vi "HDI-BBM Start Position Verify.vi"() -> ()   [LabVIEW 2011]
uses:
  Shared Components/Config Manager Class/Type Definitions/Part Type.ctl
  Shared Components/WorkTable Class/Type Definitions/Worktable_Mode.ctl
  Shared Components/Gantry Class/Gantry Class.lvclass
  Shared Components/WorkTable Class/WorkTable Class.lvclass
  Shared Components/Vec3d Class/Vec3d Class.lvclass
  Shared Components/Config Manager Class/Config Manager Class.lvclass
panel:
  in  "Worktable Mode":T1=enum."Gluing"
  in  "Part Type":T2
  in  "Chuck":i32
  in  "Quit":bool
  out "Current fiducial":string
  out "error out":errorcluster
  out "preview":T3(plugin-control)
  out "Current Position":cluster{"X":dbl, "Y":dbl, "Z":dbl}
  in  "Slot":i32
  in  "Next":bool
  in  "Config Folder":path=path "C:/Users/Husker/Desktop/gantry/Config"
  # "Set this to the appropriate slot number(0-3) before running"
  # "Set this to the appropriate chuck number(0-4) before running"
  # "Press this button to go to \nnext fiducial"
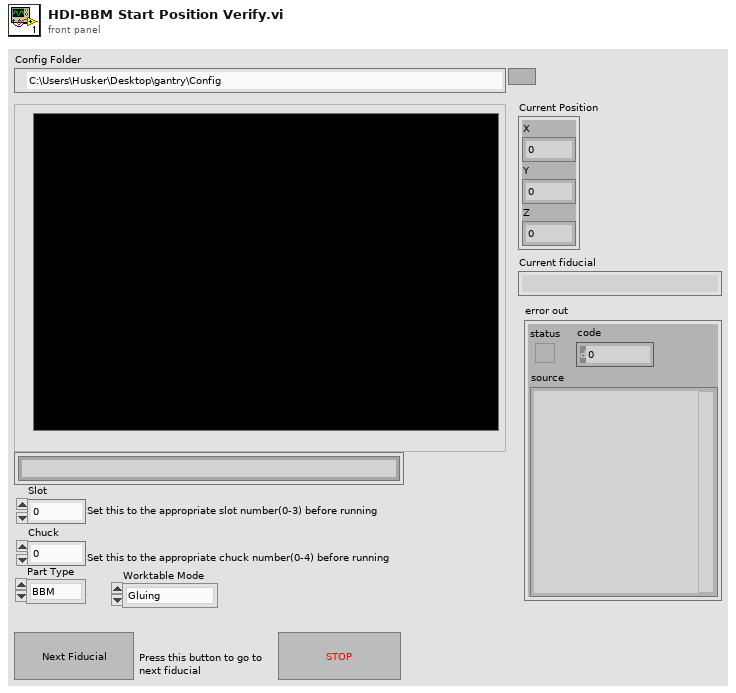
[diagram p1: front panel]
types:
  T1 = typedef "Worktable_Mode.ctl" = enum16{"Encapsulation", "Gluing"}
  T2 = typedef "Part Type.ctl" = enum16{"BBM", "HDI", "BARE HDI", "GLUERESERVOIR", "STAMP_1", "STAMP_2", "STAMP_3", "STAMP_4", "STAMP_5", "WEIGHT_1", "WEIGHT_2", "WEIGHT_3", "WEIGHT_4", "WEIGHT_5", "WEIGHT_6", "WEIGHT_7", "WEIGHT_8", "PICKER_TOOL", "GRABER_TOOL"}
  T3 = typedef "IMAQ Image.ctl" = refnum<image>
  T4 = typedef "Image Type" = u32
  T5 = typedef "Fiducial Type.ctl" = enum16{"HDI", "BBM"}
  T6 = cluster{"Feature Coordinates":refnum<class "Vec3d Class.lvclass">, "Feature Name":string}[]
  T7 = cluster{"Feature Coordinates":refnum<class "Vec3d Class.lvclass">, "Feature Name":string}
  T8 = typedef "Worktable_Module Slot.ctl" = cluster{"Slot State":enum16{"Empty", "Bare HDI", "Unglued", "Stamped", "PartOnTop", "Weighted", "Unpotted", "Potted"}, "BBM Type":enum16{"None", "BBM", "GlassSlide"}, "HDI Type":enum16{"None", "HDI", "Polyimide"}, "Vacuum Channel":u8, "Location/Orientation BBM":T9, "Location/Orientation HDI":T9, "S/N":string}
  T9 = typedef "Position_Orientation.ctl" = cluster{"Center":refnum<class "Vec3d Class.lvclass">, "Orientation":refnum<class "Orient3d Class.lvclass">}
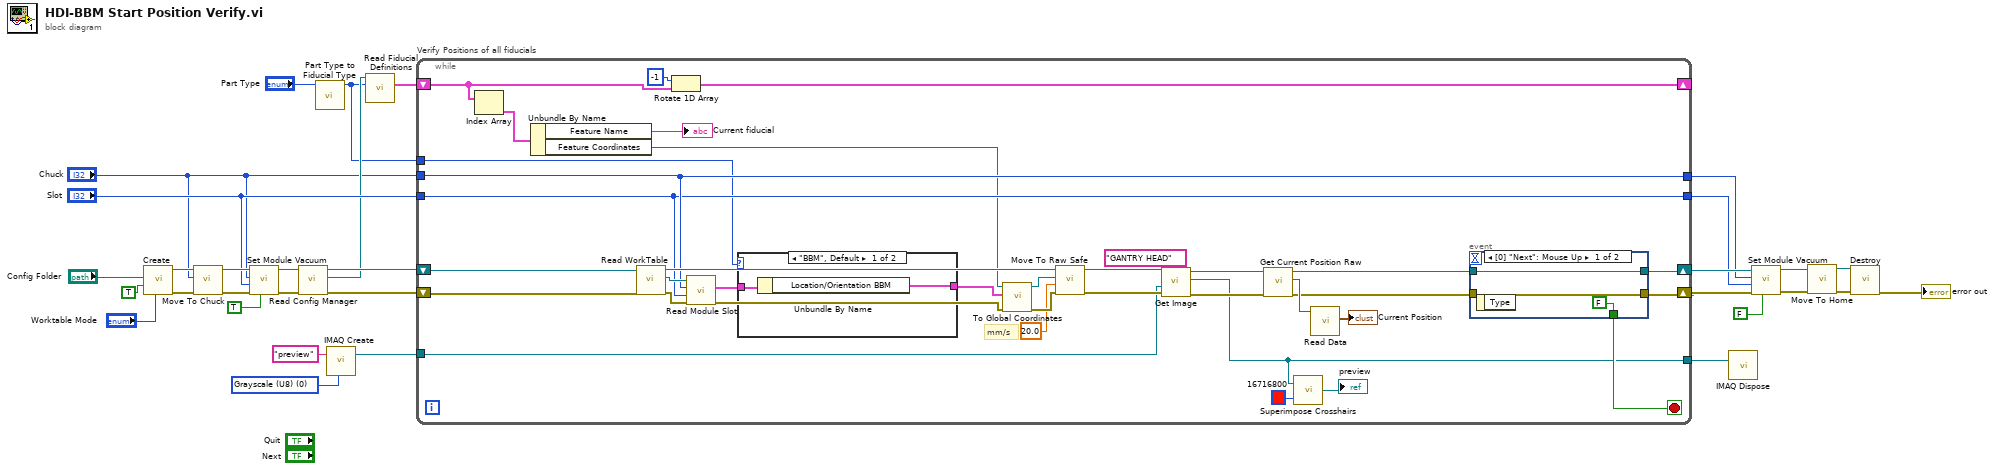
[diagram p0: block diagram]
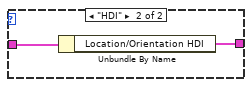
[diagram p2: hidden frame]
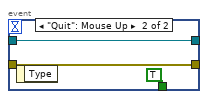
[diagram p3: hidden frame]
diagram:
  w29 = T4 0 items=["Grayscale (U8)", "Grayscale (I16)", "Grayscale (SGL)", "Complex (CSG)", "RGB (U32)", "HSL (U32)", "RGB (U64)", "Grayscale (U16)"] ("Image Type")
  n1 = call "Create.vi"("Worktable Mode"="Worktable Mode", "HOME?"=TRUE, "Config Folder"="Config Folder") -> ("error out"=w26:errorcluster, "Gantry out"=w24:refnum<class "Gantry Class.lvclass">)  [unwired: 7 in]
  n2 = call-dynamic "Move To Chuck.vi"("error in"=w26, "Chuck"="Chuck", "Gantry in"=w24) -> ("error out"=w25:errorcluster, "Gantry out"=w23:refnum<class "Gantry Class.lvclass">)  [unwired: 7 in]
  n3 = call-dynamic "Set Module Vacuum.vi"("On/Off"=TRUE, "error in"=w25, "Slot Number"="Slot", "Chuck Number"="Chuck", "Gantry in"=w23) -> ("error out"=w8:errorcluster, "Gantry out"=w9:refnum<class "Gantry Class.lvclass">)  [unwired: 5 in]
  n4 = call-dynamic "Read Config Manager.vi"("error in"=w8, "Gantry in"=w9) -> ("error out"=w6:errorcluster, "Config Manager"=w5:refnum<class "Config Manager Class.lvclass">, "Gantry out"=w7:refnum<class "Gantry Class.lvclass">)  [unwired: 7 in]
  n5 = call "Part Type to Fiducial Type.vi"("Part Type"="Part Type") -> ("Fiducial Type"=w3:T5)  [unwired: 9 in, 1 out]
  n6 = call "IMAQ Create"("Image Name"="preview", "Image Type"=w29) -> ("New Image"=w27:T3)  [unwired: 3 in, 1 out]
  n7 = call "Read Fiducial Definitions.vi"("Fiducial Type"=w3, "Config Manager in"=w5) -> ("Feature Definitions"=w4:T6)  [unwired: 7 in, 2 out]
  n8 = while "Verify Positions of all fiducials" {
    shift-right: [w48] -> w21
    shift-left: w7 -> [w36]
    shift-right: [w46] -> w20
    shift-left: w6 -> [w35]
    tunnel: w27 -> [w42]
    shift-right: [w67] -> _
    shift-left: w4 -> [w66]
    tunnel: "Slot" -> [w39]
    tunnel: [w41] -> w13
    tunnel: "Chuck" -> [w40]
    tunnel: [w40] -> w12
    tunnel: [w39] -> w11
    tunnel: w3 -> [w33]
    stop <- w44 stop-if-true
    (unwired) "GANTRY HEAD" ("Camera Name")
    # "mm/s"
    n9 = Index Array(array=w66) -> (element=w38:T7)  [unwired: 1 in]
    n10 = Unbundle By Name(w38) -> ("Feature Name"=→"Current fiducial":string, "Feature Coordinates"=w34:refnum<class "Vec3d Class.lvclass">)
    n11 = call-dynamic "Read WorkTable.vi"("error in"=w35, "Gantry Class in"=w36) -> ("error out"=w58:errorcluster, "WorkTable Class.lvclass"=w57:refnum<class "WorkTable Class.lvclass">, "Gantry Class out"=w53:refnum<class "Gantry Class.lvclass">)  [unwired: 7 in]
    n12 = Rotate 1D Array(1:w66, 2:-1 ("n")) -> (0:w67:T6)
    n13 = call-dynamic "Read Module Slot.vi"("error in"=w58, "slot"=w39, "chuck"=w40, "WorkTable in"=w57) -> ("error out"=w54:errorcluster, "Module Slot"=w56:T8)  [unwired: 5 in, 1 out]
    n14 = case shown="\"BBM\", Default" w33 {
      tunnel: w56 -> [w69 w71]
      tunnel: [w68 w70] -> w55
      frame "BBM", Default {
        n15 = Unbundle By Name(w69) -> ("Location/Orientation BBM"=w68:T9)
      }
      frame "HDI" {
        n16 = Unbundle By Name(w71) -> ("Location/Orientation HDI"=w70:T9)
      }
    }
    n17 = call "To Global Coordinates.vi"("error in"=w54, "Center/Orientation"=w55, "Local Coordinates"=w34) -> ("error out"=w51:errorcluster, "Global Coordinates"=w49:refnum<class "Vec3d Class.lvclass">)  [unwired: 7 in]
    n18 = call-dynamic "Move To Raw Safe.vi"("error in"=w51, "Speed(mm/s)"=20.0 ("Speed"), "Destination"=w49, "Gantry in"=w53) -> ("error out"=w50:errorcluster, "Gantry out"=w52:refnum<class "Gantry Class.lvclass">)  [unwired: 6 in]
    n19 = call-dynamic "Get Image.vi"("error in"=w50, "Image In"=w42, "Gantry in"=w52) -> ("error out"=w63:errorcluster, "Image Out"=w41:T3, "Gantry out"=w64:refnum<class "Gantry Class.lvclass">)  [unwired: 5 in, 1 out]
    n20 = call-dynamic "Get Current Position Raw.vi"("error in"=w63, "Gantry in"=w64) -> ("error out"=w45:errorcluster, "Vec3d Class out"=w62:refnum<class "Vec3d Class.lvclass">, "Gantry out"=w47:refnum<class "Gantry Class.lvclass">)  [unwired: 7 in]
    n21 = call "Superimpose Crosshairs.vi"("Grid Line Color"=u32 16716800, "Refnum in"=w41) -> ("Refnum out"=→"preview":T3)
    n22 = call-dynamic "Read Data.vi"("Vec3d Class in"=w62) -> ("Data"=→"Current Position":cluster{"X":dbl, "Y":dbl, "Z":dbl})  [unwired: 8 in, 2 out]
    n23 = event shown="[0] \"Next\": Mouse Up" {
      selector: _ -> [_ _]
      dyn-events: _ -> [_ _]
      timeout: _ -> [_ _]
      tunnel: [w74 w77] -> w48
      tunnel: w47 -> [w74 w77]
      tunnel: [w73 w76] -> w46
      tunnel: w45 -> [w73 w76]
      tunnel: [FALSE TRUE] -> w44
      event "Next": Mouse Up {
        n24 = event-data() -> ()  [unwired: 1 in, 1 out]
      }
      event "Quit": Mouse Up {
        n25 = event-data() -> ()  [unwired: 1 in, 1 out]
      }
    }
  }
  n26 = call "IMAQ Dispose"("Image"=w13) -> ()  [unwired: 5 in, 1 out]
  n27 = call-dynamic "Set Module Vacuum.vi"("On/Off"=FALSE, "error in"=w20, "Slot Number"=w11, "Chuck Number"=w12, "Gantry in"=w21) -> ("error out"=w15:errorcluster, "Gantry out"=w17:refnum<class "Gantry Class.lvclass">)  [unwired: 5 in]
  n28 = call-dynamic "Move To Home.vi"("error in"=w15, "Gantry in"=w17) -> ("error out"=w14:errorcluster, "Gantry out"=w16:refnum<class "Gantry Class.lvclass">)  [unwired: 8 in]
  n29 = call "Destroy.vi"("error in"=w14, "Gantry Class in"=w16) -> ("error out"=→"error out":errorcluster)  [unwired: 9 in]
